vi "Find scale factor from file name.vi"(0 "Wave File Path - READ":path) -> (14 "Scale Factor":dbl, 16 "Unit":string)   [LabVIEW 2022 SP3, in "WaveFile.lvclass"]
doc: "This vi decode the file name and tries to find the scaling factor and unit of the signals."
uses:
  WaveFile.lvclass
panel:
  out "array":string[](array[string])
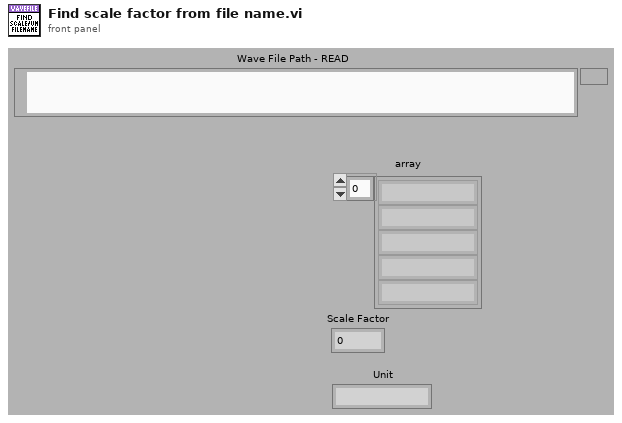
[diagram p1: front panel]
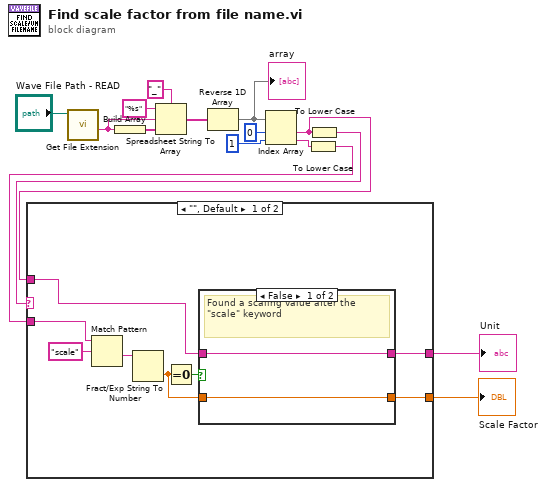
[diagram p0: block diagram]
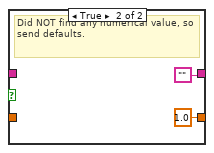
[diagram p2: hidden frame]
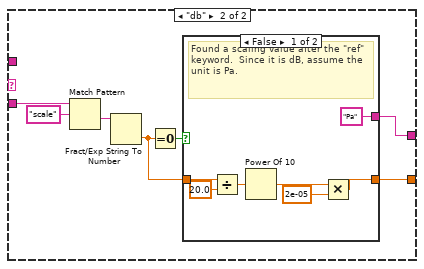
[diagram p3: hidden frame]
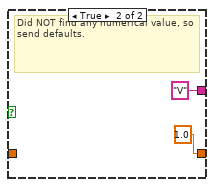
[diagram p4: hidden frame]
diagram:
  n1 = call <vilib>:"Get File Extension.vi"("file"="Wave File Path - READ") -> ("filename without extension"=w11:string)  [unwired: 6 in, 4 out]
  n2 = Build Array(w11) -> (w14:string[])
  n3 = Spreadsheet String To Array(delimiter (Tab)="_", format string="%s", spreadsheet string=w11, array type (2D Dbl)=w14) -> (array=w10:string[])
  n4 = Reverse 1D Array(array=w10) -> (reversed array=w8:string[])
  "array" <- w8
  n5 = Index Array(array=w8, index #1=0 ("index"), index #2=1 ("index")) -> (element #1=w1:string, element #2=w5:string)
  n6 = To Lower Case(string=w5) -> (all lower case string=w4:string)
  n7 = To Lower Case(string=w1) -> (all lower case string=w6:string)
  n8 = case shown="\"\", Default" w6 {
    tunnel: w4 -> [w16 w32]
    tunnel: [w23 w28] -> w3
    tunnel: [w22 w29] -> w2
    tunnel: w1 -> [w21 _]
    frame "", Default {
      n9 = Match Pattern(string=w16, regular expression="scale") -> (after substring=w19:string)  [unwired: 1 in, 3 out]
      n10 = Fract/Exp String To Number(string=w19) -> (number=w17:dbl)  [unwired: 3 in, 1 out]
      n11 = Equal To 0?(x=w17) -> (x = 0?=w18:bool)
      n12 = case shown="False" w18 {
        tunnel: [w25 1.0 ("t")] -> w23
        tunnel: w17 -> [w25 _]
        tunnel: [w24 ""] -> w22
        tunnel: w21 -> [w24 _]
        frame False {
          # "Found a scaling value after the \"scale\" keyword"
        }
        frame True {
          # "Did NOT find any numerical value, so send defaults."
        }
      }
    }
    frame "db" {
      n13 = Match Pattern(string=w32, regular expression="scale") -> (after substring=w33:string)  [unwired: 1 in, 3 out]
      n14 = Fract/Exp String To Number(string=w33) -> (number=w31:dbl)  [unwired: 3 in, 1 out]
      n15 = Equal To 0?(x=w31) -> (x = 0?=w30:bool)
      n16 = case shown="False" w30 {
        tunnel: [w35 1.0 ("t")] -> w28
        tunnel: w31 -> [w40 _]
        tunnel: ["Pa" "V"] -> w29
        frame False {
          # "Found a scaling value after the \"ref\" keyword.  Since it is dB, assume the unit is Pa."
          n17 = Divide(x=w40, y=20.0) -> (x/y=w38:dbl)
          n18 = Power Of 10(x=w38) -> (10^x=w37:dbl)
          n19 = Multiply(x=w37, y=2e-05) -> (x*y=w35:dbl)
        }
        frame True {
          # "Did NOT find any numerical value, so send defaults."
        }
      }
    }
  }
  "Scale Factor" <- w3
  "Unit" <- w2
